vi "Barometer_Calibration.vi"() -> ()   [LabVIEW 2012]
panel:
  out "Barometer sea level [hPa]":dbl format="%.1f"
  out "Offset stat. altitude [m]":dbl format="%.1f"
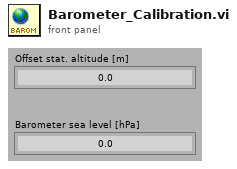
[diagram p1: front panel]
diagram:
